vi "TestReport.vi"(7 "reslut":bool, 8 "error in":errorcluster, 9 "Items out":string[][](array[string]), 11 "SN":string) -> (0 "error out":errorcluster)   [LabVIEW 2013]
uses:
  SubVi/Global constant.vi
panel:
  out "error out 2":errorcluster
  in  "error in 2":errorcluster
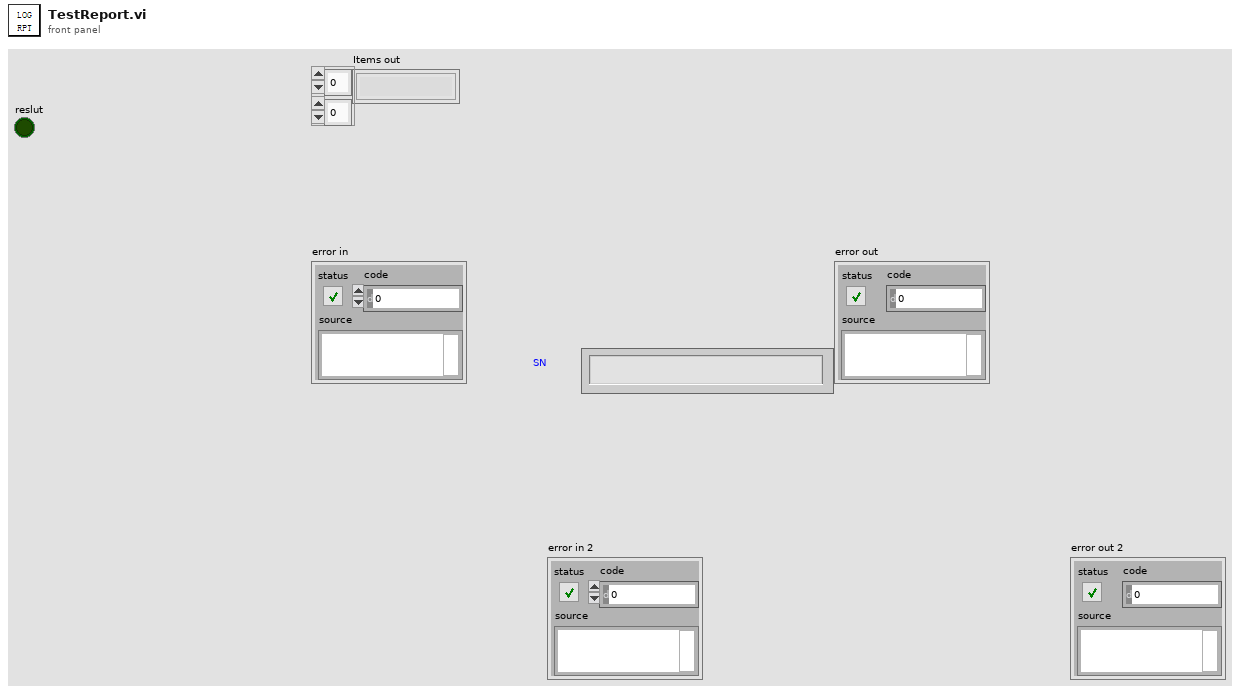
[diagram p1: front panel]
types:
  T1 = enum16{"open", "replace", "create", "open or create", "replace or create", "replace or create with confirmation"}
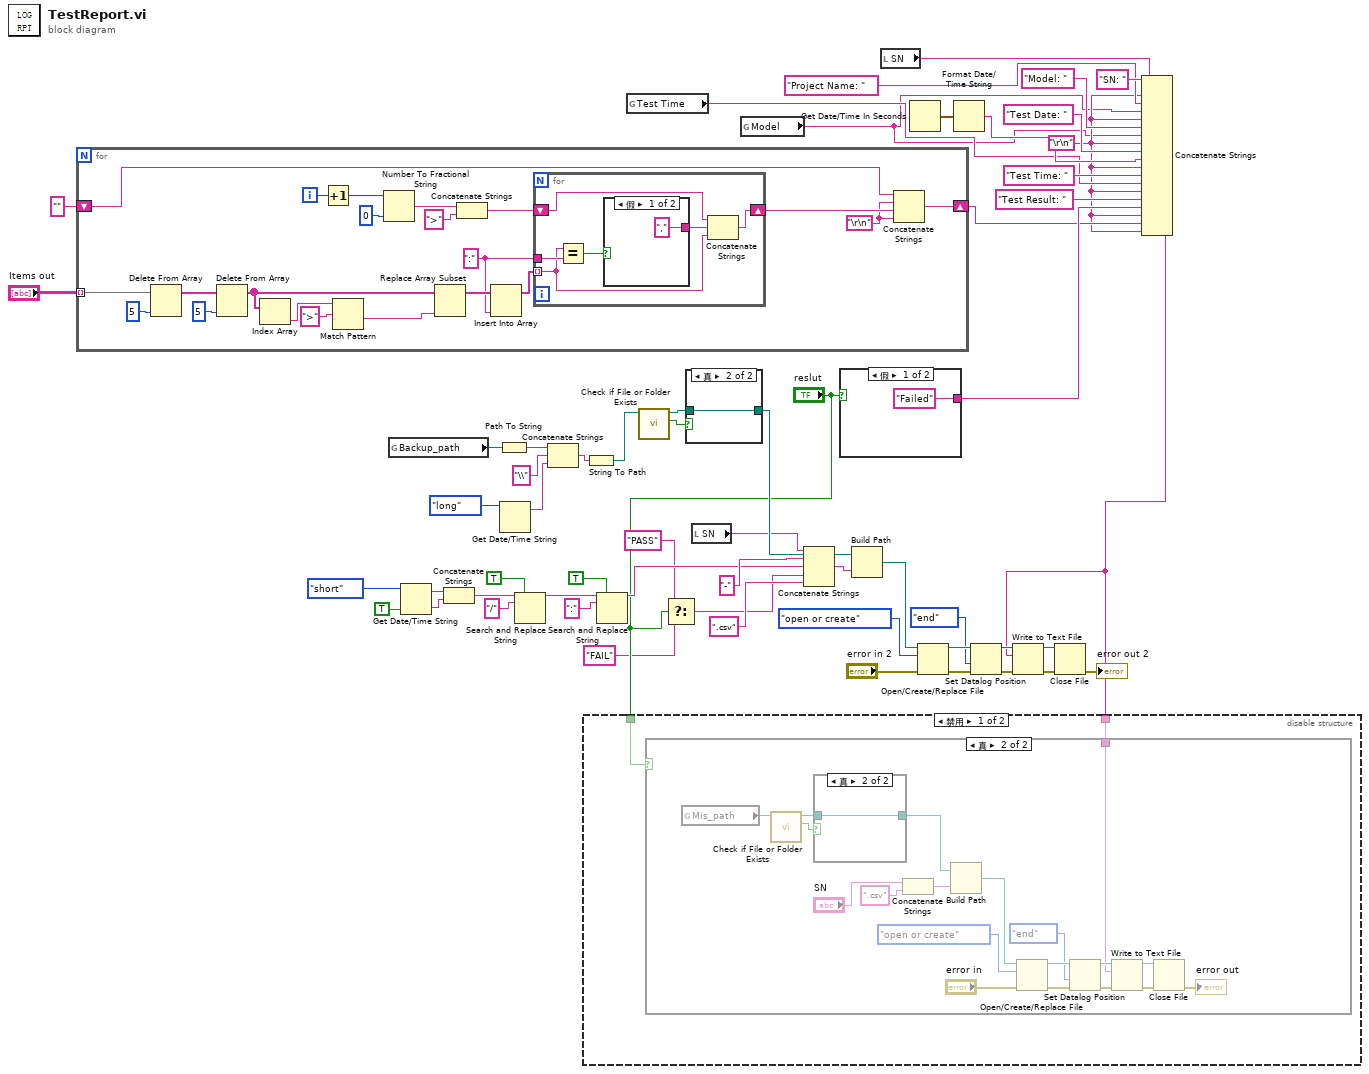
[diagram p0: block diagram]
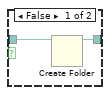
[diagram p3: hidden frame]
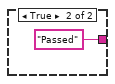
[diagram p5: hidden frame]
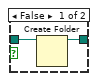
[diagram p6: hidden frame]
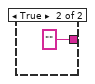
[diagram p7: hidden frame]
diagram:
  w35 = "\r\n"
  n1 = for {
    tunnel: "Items out" -> [w60] mode=indexing
    shift-right: [w72] -> w36
    shift-left: "" -> [w71]
    i -> [w78]
    w61 = ":" ("new element/subarray")
    w69 = "\r\n"
    n2 = Delete From Array(array=w60, index=5) -> (array with subset deleted=w59:string[])  [unwired: 1 in, 1 out]
    n3 = Delete From Array(array=w59, index=5) -> (array with subset deleted=w58:string[])  [unwired: 1 in, 1 out]
    n4 = Index Array(array=w58) -> (element=w66:string)  [unwired: 1 in]
    n5 = Increment(x=w78) -> (x+1=w77:i32)
    n6 = Match Pattern(string=w66, regular expression=">") -> (after substring=w65:string)  [unwired: 1 in, 3 out]
    n7 = Number To Fractional String(number=w77, precision (6)=i16 0) -> (F-format string=w76:string)  [unwired: 2 in]
    n8 = Replace Array Subset(array=w58, new element=w65) -> (w63:string[])  [unwired: 1 in]
    n9 = Concatenate Strings(w76, ">") -> (w74:string)
    n10 = Insert Into Array(array=w63, new element=w61) -> (w62:string[])  [unwired: 1 in]
    n11 = for {
      shift-right: [w83] -> w70
      shift-left: w74 -> [w84]
      tunnel: w62 -> [w81] mode=indexing
      tunnel: w61 -> [w82]
      n12 = Equal?(x=w81, y=w82) -> (x = y?=w80:bool)
      n13 = case shown="假" w80 {
        tunnel: ["," ("string") ""] -> w79
        frame False {
        }
        frame True {
        }
      }
      n14 = Concatenate Strings(w84, w79, w81) -> (w83:string)
    }
    n15 = Concatenate Strings(w71, w69, w70, w69) -> (w72:string)
  }
  n16 = global read "Global constant.vi" "Backup_path"() -> (w34:path)
  n17 = Get Date/Time String(date format (0)=enum16{"short", "long", "abbreviated"}."short", want seconds? (F)=TRUE) -> (date string=w15:string, time string=w14:string)  [unwired: 1 in]
  n18 = Concatenate Strings(w15, w14) -> (w13:string)
  n19 = Path To String(path=w34) -> (string=w48:string)
  n20 = Get Date/Time String(date format (0)=enum16{"short", "long", "abbreviated"}."long") -> (date string=w54:string)  [unwired: 2 in, 1 out]
  n21 = Search and Replace String(replace all?=TRUE ("replace all? (F)"), input string=w13, search string="/") -> (result string=w8:string)  [unwired: 5 in, 3 out]
  n22 = Concatenate Strings(w48, "\\", w54) -> (w53:string)
  n23 = String To Path(string=w53) -> (path=w52:path)
  n24 = Search and Replace String(replace all?=TRUE ("replace all? (F)"), input string=w8, search string=":") -> (result string=w7:string)  [unwired: 5 in, 3 out]
  n25 = global read "Global constant.vi" "Test Time"() -> (w39:string)
  n26 = call <vilib>:"Check if File or Folder Exists.vi"("path"=w52) -> ("file or folder exists?"=w51:bool, "dup path"=w50:path)  [unwired: 8 in, 1 out]
  n27 = Select(t="PASS" ("string"), s="reslut", f="FAIL" ("string")) -> (s? t:f=w3:string)
  n28 = case shown="真" w51 {
    tunnel: w50 -> [w88 w89]
    tunnel: [w87 w89] -> w20
    frame False {
      n29 = Create Folder(path (use dialog)=w88) -> (created path=w87:path)  [unwired: 2 in, 2 out]
    }
    frame True {
    }
  }
  n30 = local read "SN"() -> (w19:string)
  n31 = global read "Global constant.vi" "Model"() -> (w6:string)
  n32 = Concatenate Strings(w19, "-" ("string"), w7, w3, ".csv" ("string")) -> (w24:string)
  n33 = case shown="假" "reslut" {
    tunnel: ["Failed" "Passed"] -> w37
    frame False {
    }
    frame True {
    }
  }
  n34 = Build Path(base path=w20, name or relative path=w24) -> (appended path=w33:path)
  n35 = local read "SN"() -> (w45:string)
  n36 = Get Date/Time In Seconds() -> (seconds since 1Jan1904=w49:timestamp)
  n37 = Open/Create/Replace File(file path (use dialog)=w33, error in="error in 2", operation (0:open)=T1."open or create") -> (refnum out=w30:refnum<file>, error out=w31:errorcluster)  [unwired: 3 in, 1 out]
  n38 = Format Date/Time String(seconds (now)=w49) -> (date/time string=w41:string)  [unwired: 2 in]
  n39 = Set Datalog Position(4:w31, 5:enum16{"start", "end", "current"}."end" ("from (0:start)"), 7:w30) -> (0:w27:errorcluster, 3:w28:refnum<file>)  [unwired: 1 in]
  n40 = Concatenate Strings("SN: " ("string"), w45, w35, "Project Name: " ("string"), w6, w35, "Model: " ("string"), w6, w35, "Test Date: " ("string"), w41, w35, "Test Time: " ("string"), w39, w35, "Test Result: " ("string"), w37, w35, w36, w35) -> (w21:string)
  n41 = disable-structure shown="禁用" {
    disable-tunnel: "reslut" -> [w93 _]
    disable-tunnel: w21 -> [w92 _]
    frame Disabled {
      n42 = case shown="真" w93 {
        tunnel: w92 -> [_ w103]
        frame False {
        }
        frame True {
          n43 = global read "Global constant.vi" "Mis_path"() -> (w94:path)
          n44 = call <vilib>:"Check if File or Folder Exists.vi"("path"=w94) -> ("file or folder exists?"=w97:bool, "dup path"=w96:path)  [unwired: 8 in, 1 out]
          n45 = case shown="真" w97 {
            tunnel: w96 -> [w114 w115]
            tunnel: [w113 w115] -> w95
            frame False {
              n46 = Create Folder(path (use dialog)=w114) -> (created path=w113:path)  [unwired: 2 in, 2 out]
            }
            frame True {
            }
          }
          n47 = Concatenate Strings("SN", ".csv" ("string")) -> (w101:string)
          n48 = Build Path(base path=w95, name or relative path=w101) -> (appended path=w112:path)
          n49 = Open/Create/Replace File(file path (use dialog)=w112, error in="error in", operation (0:open)=T1."open or create") -> (refnum out=w109:refnum<file>, error out=w110:errorcluster)  [unwired: 3 in, 1 out]
          n50 = Set Datalog Position(4:w110, 5:enum16{"start", "end", "current"}."end" ("from (0:start)"), 7:w109) -> (0:w106:errorcluster, 3:w107:refnum<file>)  [unwired: 1 in]
          n51 = Write to Text File(file (use dialog)=w107, text=w103, error in=w106) -> (refnum out=w104:refnum<file>, error out=w105:errorcluster)  [unwired: 1 in, 1 out]
          n52 = Close File(refnum=w104, error in=w105) -> (error out=→"error out":errorcluster)  [unwired: 1 out]
        }
      }
    }
    frame Enabled {
    }
  }
  n53 = Write to Text File(file (use dialog)=w28, text=w21, error in=w27) -> (refnum out=w25:refnum<file>, error out=w26:errorcluster)  [unwired: 1 in, 1 out]
  n54 = Close File(refnum=w25, error in=w26) -> (error out=→"error out 2":errorcluster)  [unwired: 1 out]
